vi "setUp.vi"(8 "error in (no error)":errorcluster, 11 "Test Runner in":refnum<class "Test Runner.lvclass">) -> (0 "error out":errorcluster, 3 "Test Runner out":refnum<class "Test Runner.lvclass">)   [LabVIEW 2020, in "Caraya.lvlib" / "Test Runner.lvclass"]
uses:
  Test Runner.lvclass
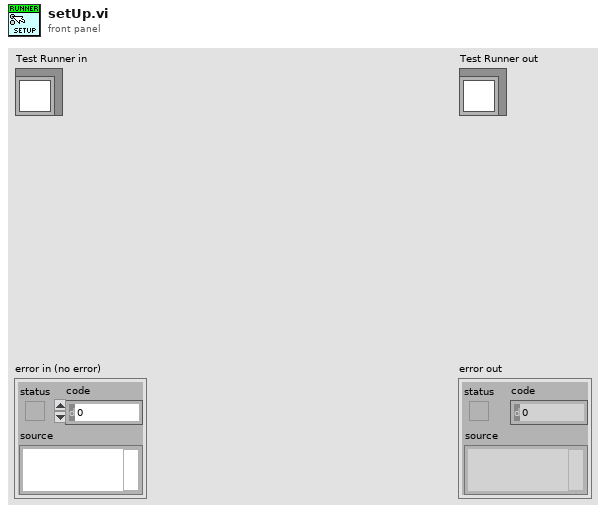
[diagram p1: front panel]
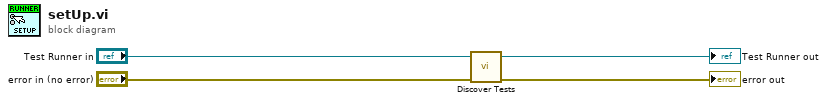
[diagram p0: block diagram]
diagram:
  n1 = call "Discover Tests.vi"("error in (no error)"="error in (no error)", "Test Runner in"="Test Runner in") -> ("error out"=→"error out":errorcluster, "Test Runner out"=→"Test Runner out":refnum<class "Test Runner.lvclass">)  [unwired: 8 in]
